vi "Auto_Change _Enum - muti-subvi.vi"() -> ()   [LabVIEW 2015]
uses:
  Enum_Edit Action.ctl
panel:
  in  "製作Form":bool
  in  "初始化歸零?":bool
  out "buttonCluster":T1
  in  "Name_data":string
  in  "Type_Buttom":enum16{"Cluster", "Control"}(ring)=enum."Control"
  in  "Type_Enum":T2(ring)=enum."Constant"
  in  "Value":string[][](array[string])
  in  "Name":string[](array[string])
  in  "檔案格式":enum16{"CSV", "Control"}(ring)
  in  "製作按鈕":bool
  out "Enum":T3
  in  "ReadFromData":bool
  in  "WriteToData":bool
  out "error out":errorcluster
  in  "初始化":bool
  in  "Data":string
  in  "結束":bool
  in  "製作Enum":bool
  in  "儲存CSV":bool
  in  "讀取CSV":bool
  in  "讀取CTL":bool
  in  "error In":errorcluster
  in  "Path":path
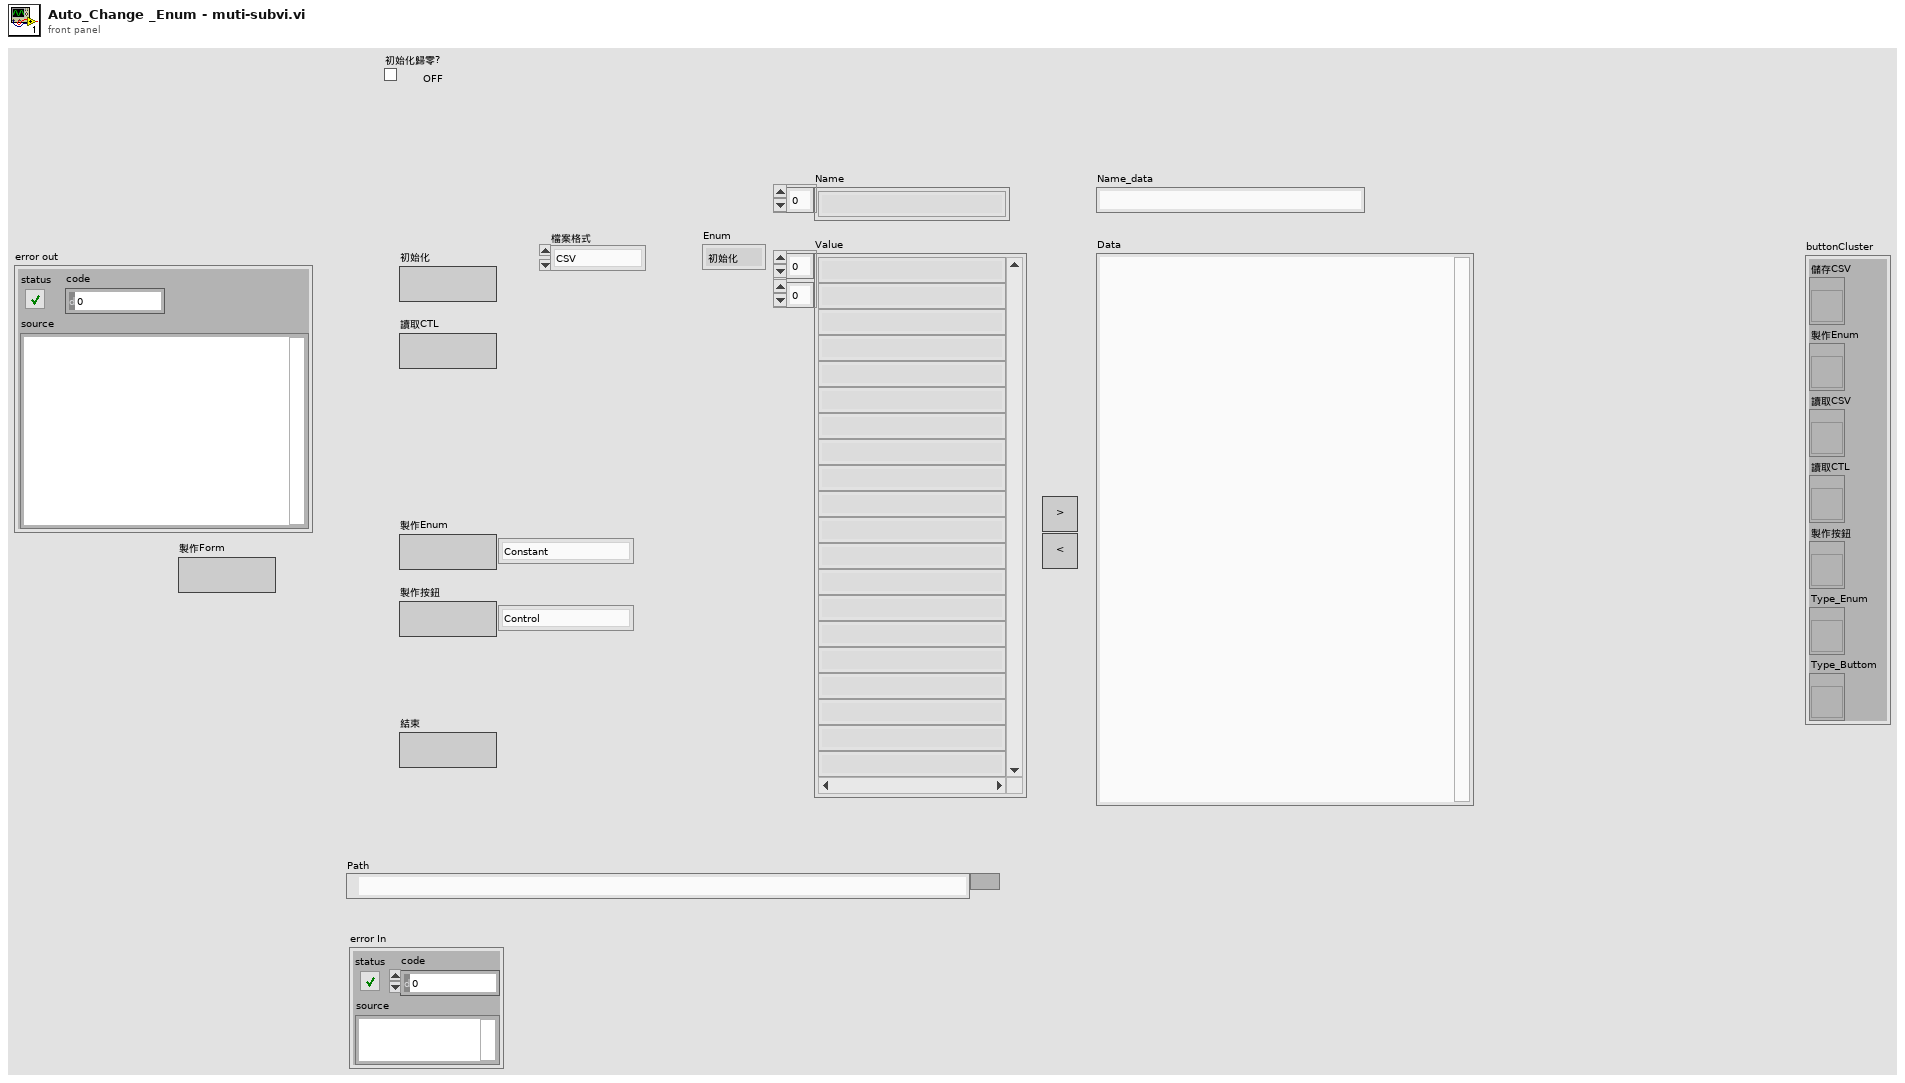
[diagram p1: front panel]
types:
  T1 = cluster{"儲存CSV":refnum<vi>, "製作Enum":refnum<vi>, "讀取CSV":refnum<vi>, "讀取CTL":refnum<vi>, "製作按鈕":refnum<vi>, "Type_Enum":refnum<vi>, "Type_Buttom":refnum<vi>}
  T2 = enum16{"Control", "Constant", "Constant(QMH)", "ClustConstant(QMH)"}
  T3 = typedef "Enum_Edit Action.ctl" = enum16{"初始化", "讀取(CSV)", "讀取(CTL)", "儲存CTL", "儲存CSV", "製作Form", "更新資料", "讀出data區", "寫入data區", "製作按鈕", "閒置", "結束"}
  T4 = cluster{"Alignment":enum32{"Left", "Right", "Hybrid", "Center", "Gravity"}, "Rules":enum32{"Strict", "Allow Wires Under Labels", "Allow Wires Under Lead Nodes", "Allow Wires Under Wide Blocks"}, "Max Heuristic Iterations":u32, "Max Simplex Iterations":u32, "Block Padding":cluster{"Horizontal":i32, "Vertical":i32}, "Wire Padding":cluster{"Horizontal":i32, "Vertical":i32}, "Auto-Tune by Topology":bool, "Fine-Tune Y Positions":bool, "Align All Controls on Left":bool, "Align All Indicators on Right":bool, "Use Array Dimension Heuristics":bool}
  T5 = enum16{"open", "replace", "create", "open or create", "replace or create", "replace or create with confirmation"}
  T6 = enum16{"讀取CTL", "讀取CSV", "儲存CSV", "製作Enum", "製作Form", "結束", "初始化", "Path", "WriteToData", "ReadFromData", "製作按鈕", "檔案格式"}
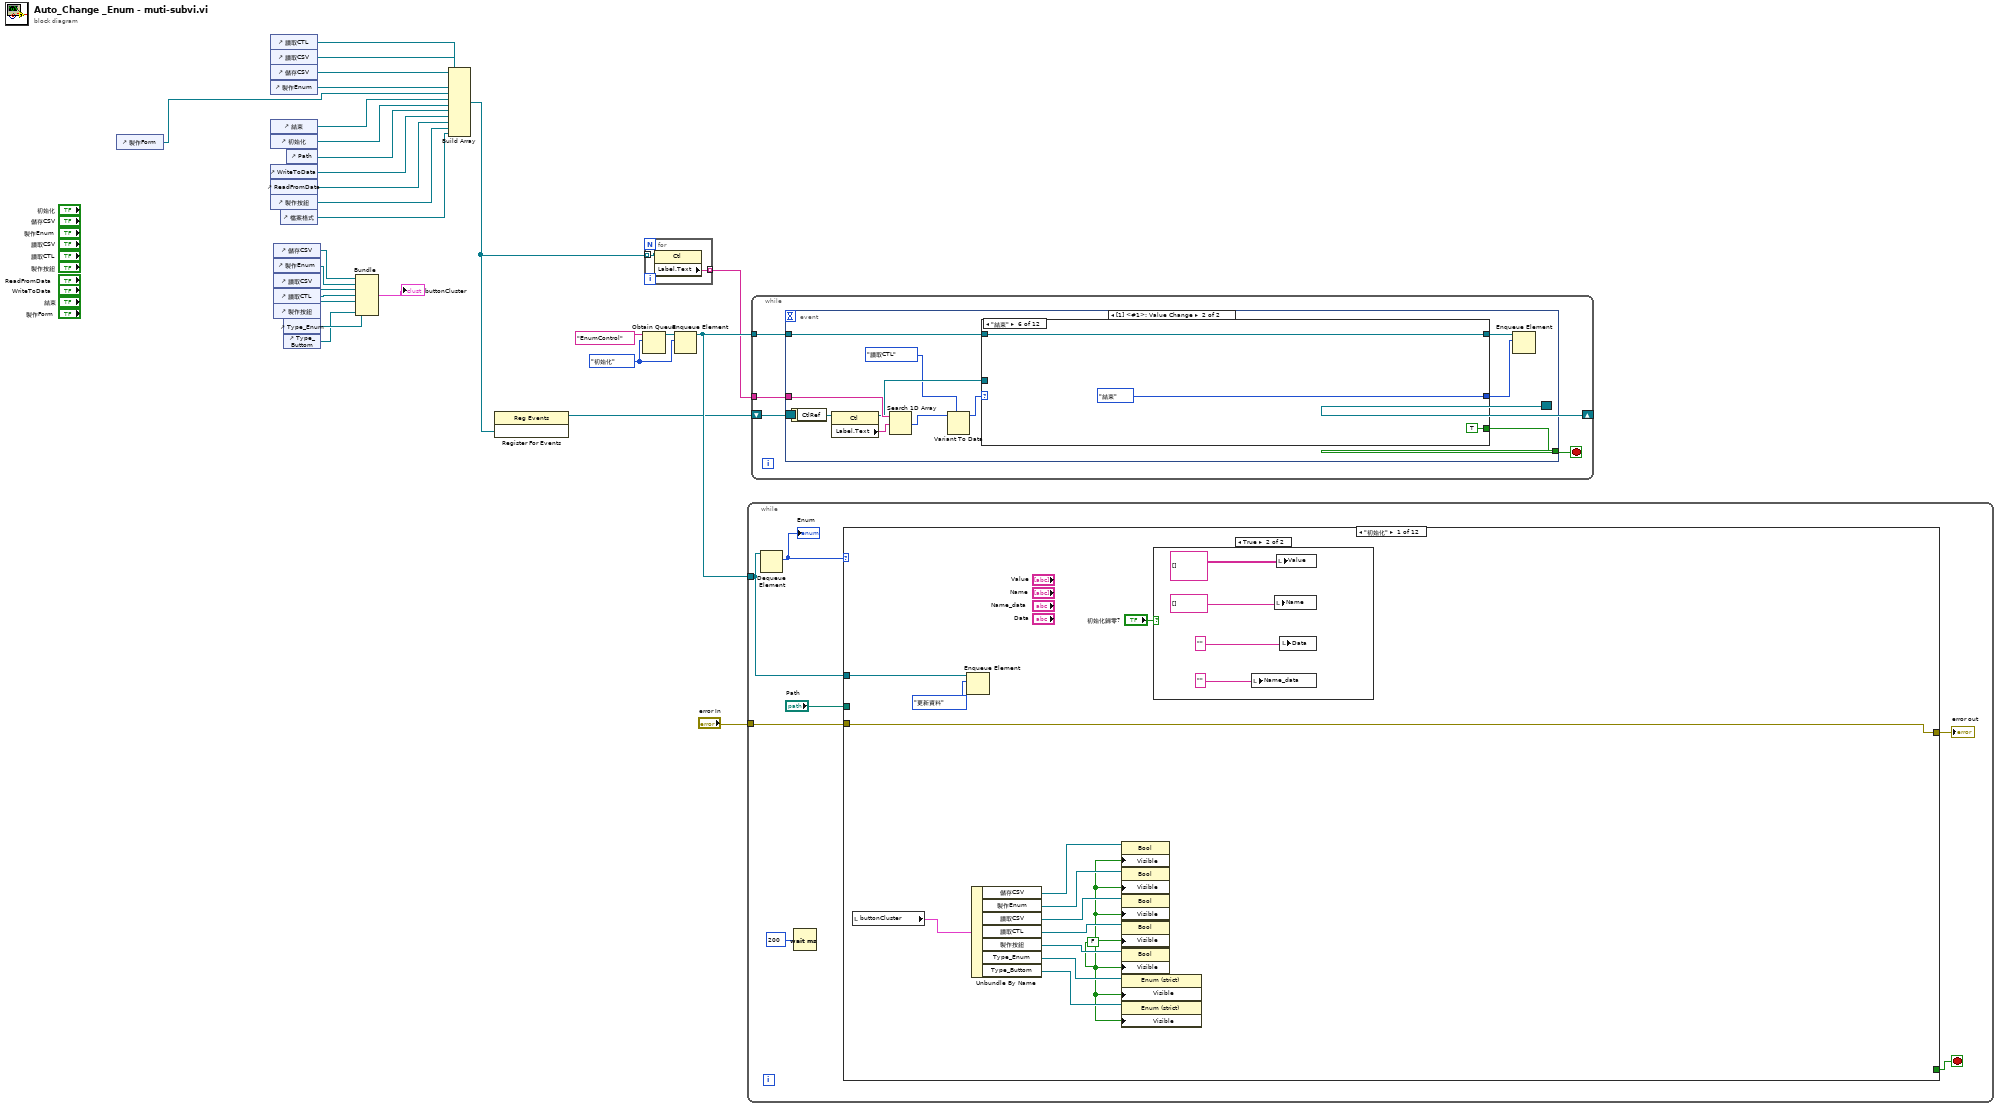
[diagram p0: block diagram]
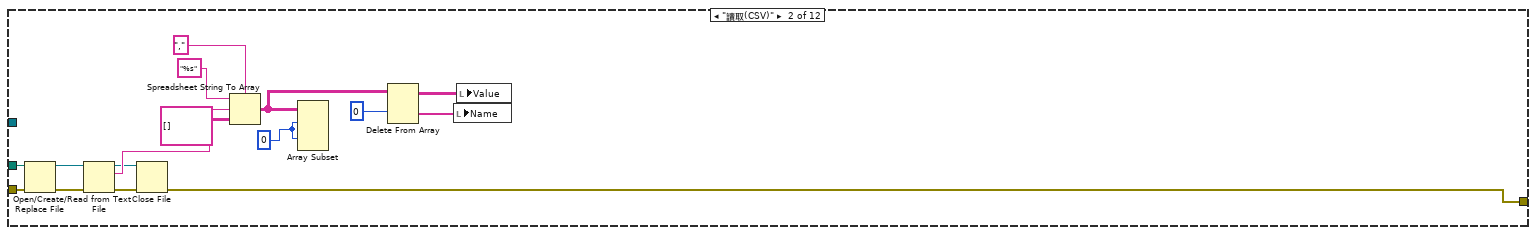
[diagram p3: hidden frame]
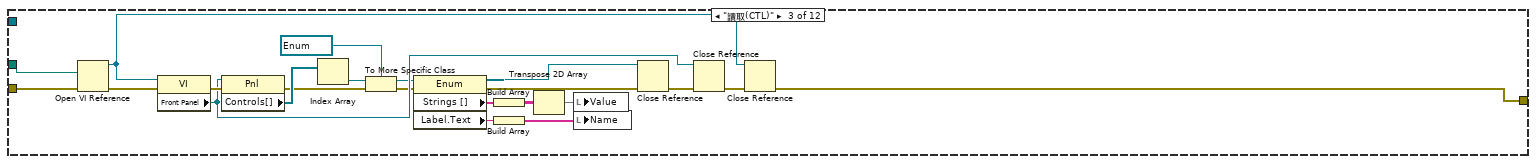
[diagram p4: hidden frame]
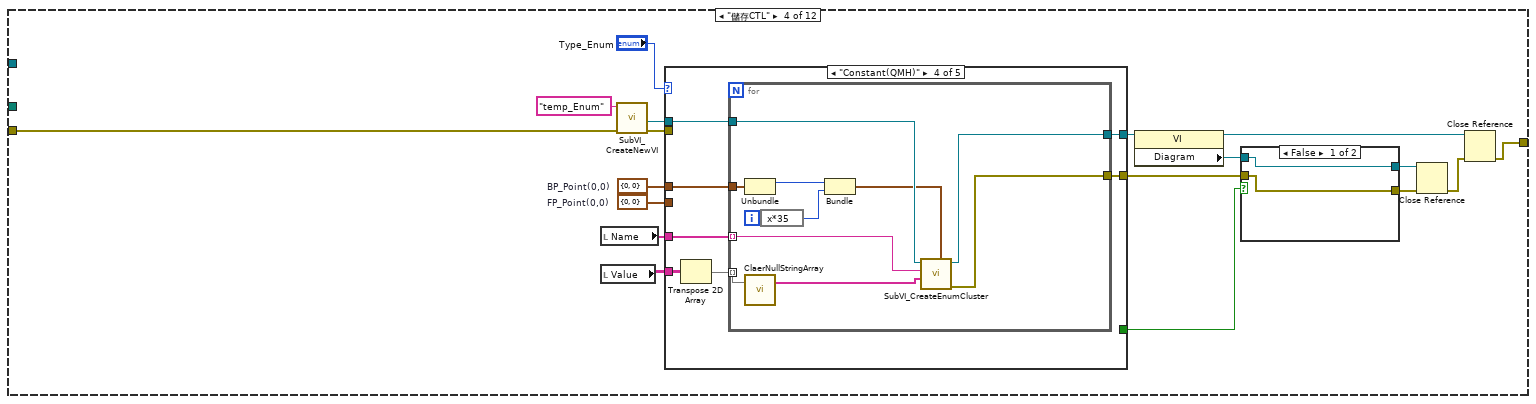
[diagram p5: hidden frame]
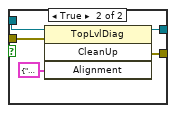
[diagram p6: hidden frame]
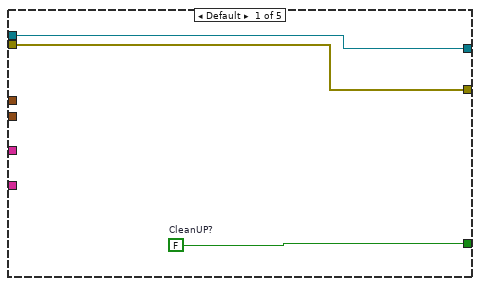
[diagram p7: hidden frame]
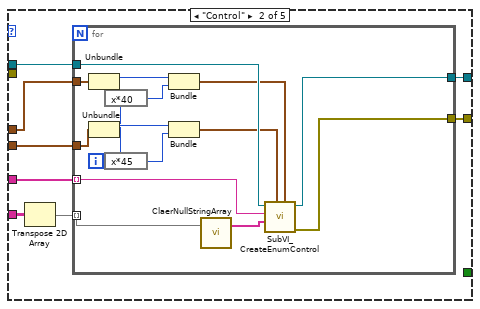
[diagram p8: hidden frame]
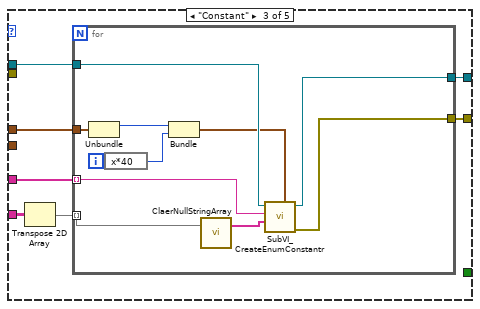
[diagram p9: hidden frame]
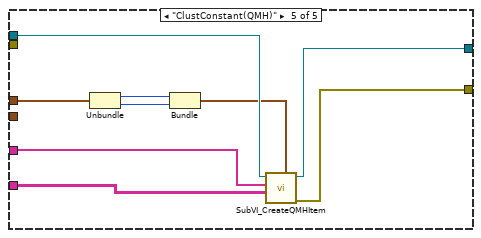
[diagram p10: hidden frame]
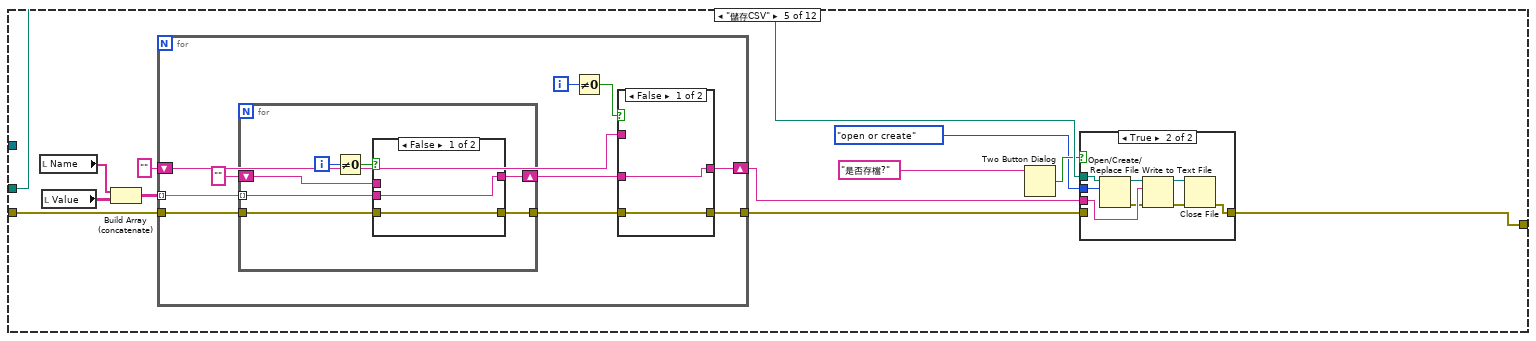
[diagram p11: hidden frame]
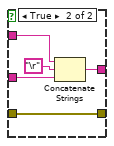
[diagram p13: hidden frame]
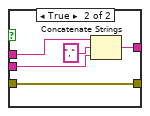
[diagram p14: hidden frame]
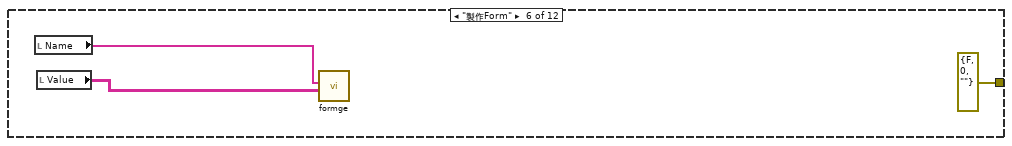
[diagram p15: hidden frame]
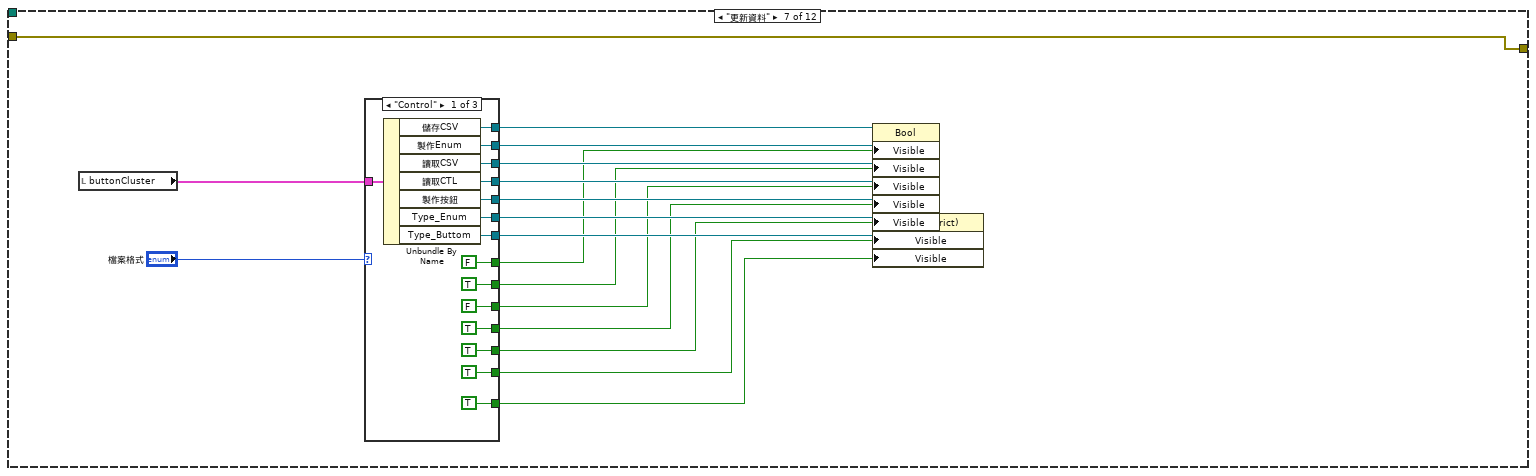
[diagram p16: hidden frame]
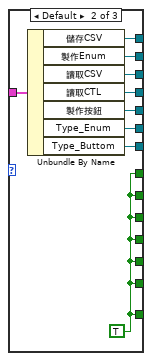
[diagram p17: hidden frame]
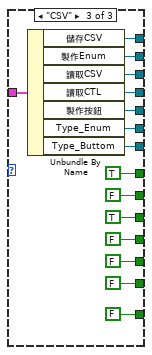
[diagram p18: hidden frame]
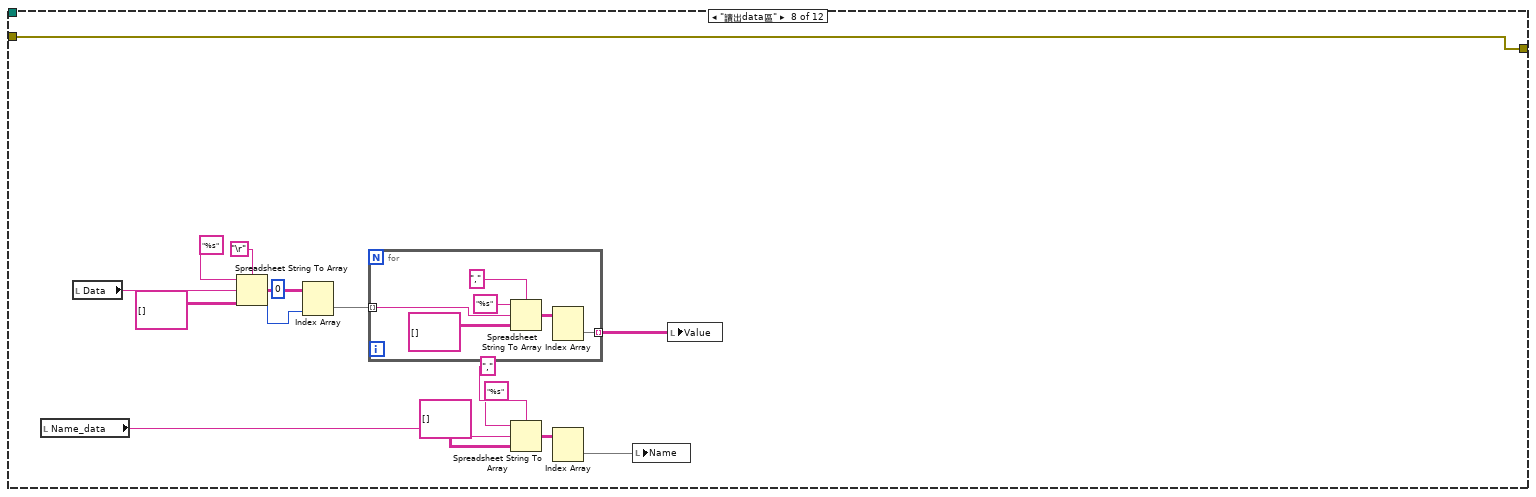
[diagram p19: hidden frame]
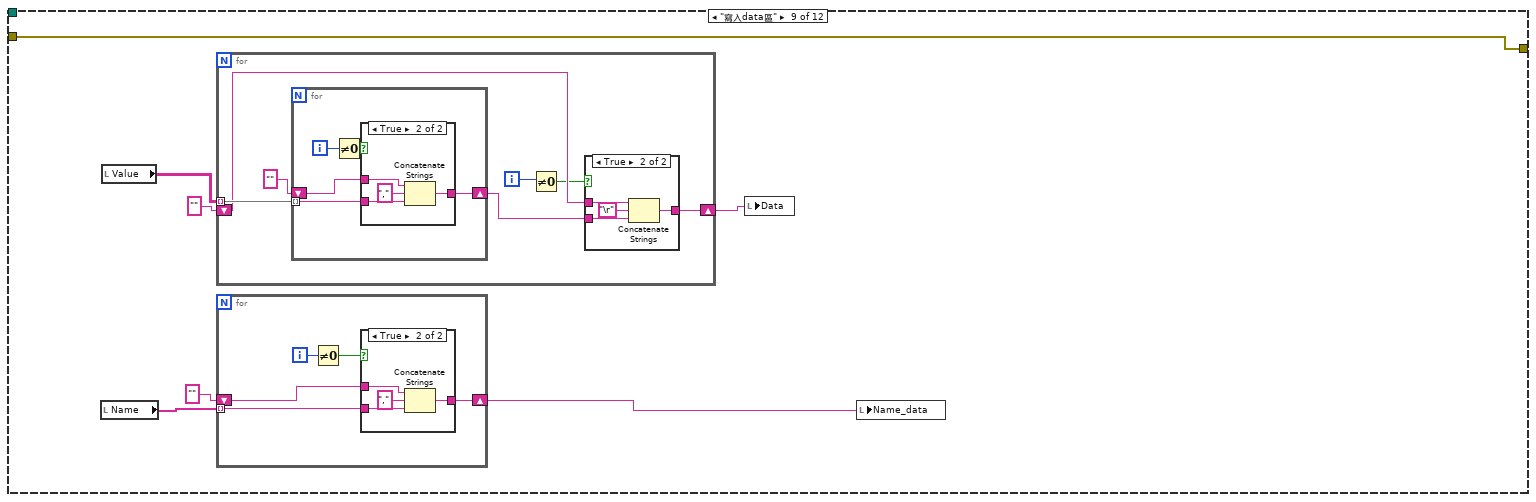
[diagram p20: hidden frame]
diagram:
  w24 = Enum_Edit_Action."初始化" ("Enum")
  n1 = control-ref of="製作Form"() -> (w2:refnum<vi>)
  n2 = control-ref of="讀取CTL"() -> (w15:refnum<vi>)
  n3 = control-ref of="讀取CSV"() -> (w14:refnum<vi>)
  n4 = control-ref of="儲存CSV"() -> (w13:refnum<vi>)
  n5 = control-ref of="製作Enum"() -> (w12:refnum<vi>)
  n6 = control-ref of="結束"() -> (w11:refnum<vi>)
  n7 = control-ref of="初始化"() -> (w10:refnum<vi>)
  n8 = control-ref of="WriteToData"() -> (w8:refnum<vi>)
  n9 = control-ref of="ReadFromData"() -> (w7:refnum<vi>)
  n10 = control-ref of="製作按鈕"() -> (w6:refnum<vi>)
  n11 = control-ref of="儲存CSV"() -> (w21:refnum<vi>)
  n12 = control-ref of="製作Enum"() -> (w16:refnum<vi>)
  n13 = control-ref of="讀取CSV"() -> (w18:refnum<vi>)
  n14 = control-ref of="讀取CTL"() -> (w20:refnum<vi>)
  n15 = control-ref of="製作按鈕"() -> (w19:refnum<vi>)
  n16 = control-ref of="檔案格式"() -> (w5:refnum<vi>)
  n17 = control-ref of="Type_Enum"() -> (w23:refnum<vi>)
  n18 = control-ref of="Type_Buttom"() -> (w17:refnum<vi>)
  n19 = control-ref of="Path"() -> (w9:refnum<vi>)
  n20 = Bundle("儲存CSV"=w21, "製作Enum"=w16, "讀取CSV"=w18, "讀取CTL"=w20, "製作按鈕"=w19, "Type_Enum"=w23, "Type_Buttom"=w17) -> (→"buttonCluster":T1)  [unwired: 1 in]
  n21 = Build Array(w15, w14, w13, w12, w2, w11, w10, w9, w8, w7, w6, w5) -> (w3:refnum<vi>[])
  n22 = register-events(w3) -> (reference out=w22:refnum<event-registration>)  [unwired: 2 in, 1 out]
  n23 = Obtain Queue(name (unnamed)="EnumControl", element data type=w24) -> (queue out=w27:refnum<queue>)  [unwired: 3 in, 2 out]
  n24 = for {
    tunnel: w3 -> [w30] mode=indexing
    tunnel: [w29] -> w1 mode=indexing
    n25 = property class="Ctl"(reference=w30) -> ("Label.Text"=w29:string)  [unwired: 1 in, 2 out]
  }
  n26 = Enqueue Element(queue=w27, element=w24) -> (queue out=w26:refnum<queue>)  [unwired: 2 in, 2 out]
  n27 = while {
    tunnel: w26 -> [w32]
    tunnel: "error In" -> [w35]
    stop <- w36 stop-if-true
    n28 = Dequeue Element(queue=w32) -> (element=w34:T3)  [unwired: 2 in, 3 out]
    "Enum" <- w34
    n29 = Wait (ms)(milliseconds to wait=u32 200) -> ()  [unwired: 1 out]
    n30 = case shown="\"初始化\"" w34 {
      tunnel: [_ _ _ _ _ _ _ _ _ _ _ TRUE] -> w36
      tunnel: w35 -> [w46 w60 w88 w94 w195 _ w260 w314 w327 w372 w440 w441]
      tunnel: [w46 w57 w79 w100 w194 errorcluster {"status"=FALSE, "code"=0, "source"=""} ("error In") w260 w314 w327 w363 w440 w441] -> w33
      tunnel: w32 -> [w43 _ _ _ _ _ _ _ _ _ _ _]
      tunnel: "Path" -> [_ w59 w72 _ w193 _ _ _ _ _ _ _]
      frame "初始化" {
        w39 = FALSE ("Visible")
        n31 = local read "buttonCluster"() -> (w45:T1)
        n32 = Enqueue Element(queue=w43, element=Enum_Edit_Action."更新資料" ("Enum")) -> ()  [unwired: 2 in, 3 out]
        n33 = Unbundle By Name(w45) -> ("儲存CSV"=w50:refnum<vi>, "製作Enum"=w49:refnum<vi>, "讀取CSV"=w48:refnum<vi>, "讀取CTL"=w47:refnum<vi>, "製作按鈕"=w44:refnum<vi>, "Type_Enum"=w41:refnum<vi>, "Type_Buttom"=w40:refnum<vi>)
        n34 = property class="Bool"(reference=w50, "Visible"=w39) -> ()  [unwired: 1 in, 2 out]
        n35 = property class="Bool"(reference=w49, "Visible"=w39) -> ()  [unwired: 1 in, 2 out]
        n36 = property class="Bool"(reference=w48, "Visible"=w39) -> ()  [unwired: 1 in, 2 out]
        n37 = property class="Bool"(reference=w47, "Visible"=w39) -> ()  [unwired: 1 in, 2 out]
        n38 = property class="Bool"(reference=w44, "Visible"=w39) -> ()  [unwired: 1 in, 2 out]
        n39 = property class="Enum (strict)"(reference=w41, "Visible"=w39) -> ()  [unwired: 1 in, 2 out]
        n40 = property class="Enum (strict)"(reference=w40, "Visible"=w39) -> ()  [unwired: 1 in, 2 out]
        n41 = case shown="True" "初始化歸零?" {
          frame False {
          }
          frame True {
            n42 = local write "Name_data"("" ("Data")) -> ()
            n43 = local write "Name"(string[] []) -> ()
            n44 = local write "Value"(string[][] []) -> ()
            n45 = local write "Data"("" ("Data")) -> ()
          }
        }
      }
      frame "讀取(CSV)" {
        w58 = 0 ("index")
        n46 = Open/Create/Replace File(file path (use dialog)=w59, error in=w60) -> (refnum out=w70:refnum<file>, error out=w63:errorcluster)  [unwired: 4 in, 1 out]
        n47 = Read from Text File(file (use dialog)=w70, error in=w63) -> (refnum out=w65:refnum<file>, text=w68:string, error out=w64:errorcluster)  [unwired: 2 in, 1 out]
        n48 = Close File(refnum=w65, error in=w64) -> (error out=w57:errorcluster)  [unwired: 1 out]
        n49 = Spreadsheet String To Array(delimiter (Tab)=",", format string="%s" ("delimiter (\\t)"), spreadsheet string=w68, array type (2D Dbl)=string[][] [] ("Array")) -> (array=w62:string[][])
        n50 = Array Subset(array=w62, index (row)=w58, index (col)=w58) -> ()  [unwired: 2 in, 1 out]
        n51 = Delete From Array(array=w62, index (row)=0) -> (deleted portion=w56:string[], array with subset deleted=w55:string[][])  [unwired: 2 in]
        n52 = local write "Name"(w56) -> ()
        n53 = local write "Value"(w55) -> ()
      }
      frame "讀取(CTL)" {
        n54 = Open VI Reference(vi path=w72, error in (no error)=w88) -> (vi reference=w71:refnum<vi>, error out=w87:errorcluster)  [unwired: 4 in]
        n55 = property class="VI"(reference=w71, error in=w87) -> (error out=w90:errorcluster, "Front Panel"=w89:refnum<vi>)  [unwired: 1 out]
        n56 = property class="Pnl"(reference=w89, error in=w90) -> (error out=w80:errorcluster, "Controls[]"=w86:refnum<vi>[])  [unwired: 1 out]
        n57 = Index Array(array=w86) -> (element=w78:refnum<vi>)  [unwired: 1 in]
        n58 = To More Specific Class(target class=refnum<vi> refnum, reference=w78, error in=w80) -> (specific class reference=w84:refnum<vi>, error out=w82:errorcluster)
        n59 = property class="Enum"(reference=w84, error in=w82) -> (reference out=w83:refnum<vi>, error out=w81:errorcluster, "Strings []"=w77:string[], "Label.Text"=w76:string)
        n60 = Build Array(w77) -> (w74:string[][])
        n61 = Build Array(w76) -> (w75:string[])
        n62 = Transpose 2D Array(2D array=w74) -> (transposed array=w73:string[][])
        n63 = local write "Value"(w73) -> ()
        n64 = local write "Name"(w75) -> ()
        n65 = Close Reference(reference=w83, error in (no error)=w81) -> (error out=w92:errorcluster)
        n66 = Close Reference(reference=w89, error in (no error)=w92) -> (error out=w91:errorcluster)
        n67 = Close Reference(reference=w71, error in (no error)=w91) -> (error out=w79:errorcluster)
      }
      frame "儲存CTL" {
        w97 = cluster{"Width":i32, "Height":i32} {"Width"=0, "Height"=0}  # FP_Point(0,0)
        w98 = cluster{"Width":i32, "Height":i32} {"Width"=0, "Height"=0}  # BP_Point(0,0)
        n68 = local read "Name"() -> (w105:string[])
        n69 = local read "Value"() -> (w110:string[][])
        n70 = call "SubVI_CreateNewVI.vi"("error in (no error)"=w94, "vi path"="temp_Enum") -> ("error out"=w95:errorcluster, "VI out"=w96:refnum<vi>)  [unwired: 8 in]
        n71 = case shown="\"Constant(QMH)\"" "Type_Enum" {
          tunnel: w110 -> [_ w125 w150 w165 w187]
          tunnel: w96 -> [w119 w126 w148 w167 w186]
          tunnel: w105 -> [_ w127 w147 w166 w188]
          tunnel: [w119 w124 w146 w164 w185] -> w104
          tunnel: [w118 w123 w145 w163 w184] -> w101
          tunnel: [w120 _ _ _ _] -> w99
          tunnel: w95 -> [w118 _ _ _ _]
          tunnel: w98 -> [_ w121 w144 w162 w182]
          tunnel: w97 -> [_ w122 _ _ _]
          frame Default {
            w120 = FALSE  # CleanUP?
          }
          frame "Control" {
            n72 = Transpose 2D Array(2D array=w125) -> (transposed array=w128:string[][])
            n73 = for {
              tunnel: w128 -> [w143] mode=indexing
              tunnel: w126 -> [w142]
              tunnel: w127 -> [w139] mode=indexing
              tunnel: [w140] -> w124
              tunnel: [w138] -> w123
              tunnel: w122 -> [w135]
              tunnel: w121 -> [w132]
              i -> [w131]
              n74 = Unbundle(w132) -> ("Width"=w134:i32)  [unwired: 1 out]
              n75 = Unbundle(w135) -> ("Width"=w136:i32)  [unwired: 1 out]
              n76 = expression code="x*40"(w131) -> (w133:i32)
              n77 = expression code="x*45"(w131) -> (w137:i32)
              n78 = Bundle("Width"=w134, w133) -> (w130:cluster{"Width":i32, i32})  [unwired: 1 in]
              n79 = Bundle("Width"=w136, w137) -> (w129:cluster{"Width":i32, i32})  [unwired: 1 in]
              n80 = call <userlib>:"ClaerNullStringArray.vi"("Array in"=w143) -> ("Array out"=w141:string[])  [unwired: 18 in]
              n81 = call "SubVI_CreateEnumControl.vi"("BP_Point(0,0)"=w130, "FP_Point(0,0)"=w129, "Value"=w141, "Name"=w139, "VI in"=w142) -> ("error out"=w138:errorcluster, "VI out"=w140:refnum<vi>)  [unwired: 5 in]
            }
          }
          frame "Constant" {
            n82 = Transpose 2D Array(2D array=w150) -> (transposed array=w149:string[][])
            n83 = for {
              tunnel: w149 -> [w161] mode=indexing
              tunnel: w148 -> [w160]
              tunnel: w147 -> [w157] mode=indexing
              tunnel: [w159] -> w146
              tunnel: [w156] -> w145
              tunnel: w144 -> [w155]
              i -> [w154]
              n84 = Unbundle(w155) -> ("Width"=w151:i32)  [unwired: 1 out]
              n85 = expression code="x*40"(w154) -> (w152:i32)
              n86 = Bundle("Width"=w151, w152) -> (w153:cluster{"Width":i32, i32})  [unwired: 1 in]
              n87 = call <userlib>:"ClaerNullStringArray.vi"("Array in"=w161) -> ("Array out"=w158:string[])  [unwired: 18 in]
              n88 = call "SubVI_CreateEnumConstantr.vi"("BP_Point(0,0)"=w153, "Value"=w158, "Name"=w157, "VI in"=w160) -> ("error out"=w156:errorcluster, "VI out"=w159:refnum<vi>)  [unwired: 6 in]
            }
          }
          frame "Constant(QMH)" {
            n89 = Transpose 2D Array(2D array=w165) -> (transposed array=w168:string[][])
            n90 = for {
              tunnel: w168 -> [w179] mode=indexing
              tunnel: w167 -> [w178]
              tunnel: w166 -> [w177] mode=indexing
              tunnel: [w175] -> w164
              tunnel: [w174] -> w163
              tunnel: w162 -> [w173]
              i -> [w172]
              n91 = Unbundle(w173) -> ("Width"=w169:i32)  [unwired: 1 out]
              n92 = call <userlib>:"ClaerNullStringArray.vi"("Array in"=w179) -> ("Array out"=w176:string[])  [unwired: 18 in]
              n93 = expression code="x*35"(w172) -> (w170:i32)
              n94 = Bundle("Width"=w169, w170) -> (w171:cluster{"Width":i32, i32})  [unwired: 1 in]
              n95 = call "SubVI_CreateEnumCluster.vi"("BP_Point(0,0)"=w171, "Data"=w176, "Name"=w177, "VI in"=w178) -> ("error out"=w174:errorcluster, "VI out"=w175:refnum<vi>)  [unwired: 5 in, 1 out]
            }
          }
          frame "ClustConstant(QMH)" {
            n96 = Unbundle(w182) -> ("Width"=w181:i32, "Height"=w183:i32)
            n97 = Bundle("Width"=w181, "Height"=w183) -> (w180:cluster{"Width":i32, "Height":i32})  [unwired: 1 in]
            n98 = call "SubVI_CreateQMHItem.vi"("BP_Point(0,0)"=w180, "Value"=w187, "Name"=w188, "VI in"=w186) -> ("error out"=w184:errorcluster, "VI out"=w185:refnum<vi>)  [unwired: 6 in]
          }
        }
        n99 = property on="Property Node" class="VI"(reference=w104) -> (reference out=w102:refnum<vi>, "Diagram"=w103:refnum<vi>)  [unwired: 1 in, 1 out]
        n100 = case shown="False" w99 {
          tunnel: [w112 w117] -> w109
          tunnel: [w111 w116] -> w108
          tunnel: w103 -> [w112 w114]
          tunnel: w101 -> [w111 w113]
          frame False {
          }
          frame True {
            n101 = invoke class="TopLvlDiag" method="CleanUp"(reference=w114, error in=w113, "Alignment"=T4 {"Alignment"=enum."Left", "Rules"=enum."Strict", "Max Heuristic Iterations"=0, "Max Simplex Iterations"=0, "Block Padding"={"Horizontal"=0, "Vertical"=0}, "Wire Padding"={"Horizontal"=0, "Vertical"=0}, "Auto-Tune by Topology"=FALSE, "Fine-Tune Y Positions"=FALSE, "Align All Controls on Left"=FALSE, "Align All Indicators on Right"=FALSE, "Use Array Dimension Heuristics"=FALSE} ("Clean Up Options")) -> (reference out=w117:refnum<vi>, error out=w116:errorcluster)  [unwired: 1 in, 2 out]
          }
        }
        n102 = Close Reference(reference=w109, error in (no error)=w108) -> (error out=w107:errorcluster)
        n103 = Close Reference(reference=w102, error in (no error)=w107) -> (error out=w100:errorcluster)
      }
      frame "儲存CSV" {
        n104 = local read "Name"() -> (w197:string[])
        n105 = local read "Value"() -> (w198:string[][])
        n106 = Build Array (concatenate)(w197, w198) -> (w196:string[][])
        n107 = for {
          tunnel: w196 -> [w219] mode=indexing
          shift-right: [w215] -> w200
          shift-left: "" -> [w216]
          tunnel: [w212] -> w199
          tunnel: w195 -> [w210]
          i -> [w214]
          n108 = for {
            tunnel: w219 -> [w233] mode=indexing
            shift-right: [w231] -> w217
            shift-left: "" -> [w232]
            tunnel: [w228] -> w211
            tunnel: w210 -> [w227]
            i -> [w230]
            n109 = Not Equal To 0?(x=w230) -> (x != 0?=w229:bool)
            n110 = case shown="False" w229 {
              tunnel: w233 -> [w235 w239]
              tunnel: w232 -> [_ w238]
              tunnel: [w235 w237] -> w231
              tunnel: [w234 w236] -> w228
              tunnel: w227 -> [w234 w236]
              frame False {
              }
              frame True {
                n111 = Concatenate Strings(w238, ",", w239) -> (w237:string)
              }
            }
          }
          n112 = Not Equal To 0?(x=w214) -> (x != 0?=w213:bool)
          n113 = case shown="False" w213 {
            tunnel: w217 -> [w221 w226]
            tunnel: w216 -> [_ w224]
            tunnel: [w221 w223] -> w215
            tunnel: [w220 w222] -> w212
            tunnel: w211 -> [w220 w222]
            frame False {
            }
            frame True {
              n114 = Concatenate Strings(w224, "\r", w226) -> (w223:string)
            }
          }
        }
        n115 = Two Button Dialog(message="是否存檔?") -> (T button?=w191:bool)  [unwired: 2 in]
        n116 = case shown="True" w191 {
          tunnel: T5."open or create" ("operation (0:open)") -> [_ w208]
          tunnel: w200 -> [_ w207]
          tunnel: [w201 w204] -> w194
          tunnel: w193 -> [_ w202]
          tunnel: w199 -> [w201 _]
          frame False {
          }
          frame True {
            n117 = Open/Create/Replace File(file path (use dialog)=w202, operation (0:open)=w208) -> (refnum out=w209:refnum<file>, error out=w203:errorcluster)  [unwired: 4 in, 1 out]
            n118 = Write to Text File(file (use dialog)=w209, text=w207, error in=w203) -> (refnum out=w205:refnum<file>, error out=w206:errorcluster)  [unwired: 1 in, 1 out]
            n119 = Close File(refnum=w205, error in=w206) -> (error out=w204:errorcluster)  [unwired: 1 out]
          }
        }
      }
      frame "製作Form" {
        n120 = local read "Name"() -> (w242:string[])
        n121 = local read "Value"() -> (w241:string[][])
        n122 = call "formge.vi"("Data"=w241, "DataName"=w242) -> ()  [unwired: 10 in]
      }
      frame "更新資料" {
        n123 = local read "buttonCluster"() -> (w247:T1)
        n124 = case shown="\"Control\"" "檔案格式" {
          tunnel: w247 -> [w268 w276 w299]
          tunnel: [w275 w284 w298] -> w259
          tunnel: [w274 w283 w297] -> w258
          tunnel: [w273 w282 w296] -> w257
          tunnel: [w272 w281 w295] -> w256
          tunnel: [w271 w280 w294] -> w255
          tunnel: [w270 w279 w293] -> w254
          tunnel: [w269 w278 w292] -> w253
          tunnel: [TRUE ("Visible") w277 FALSE ("Visible")] -> w252
          tunnel: [TRUE ("Visible") w277 FALSE ("Visible")] -> w244
          tunnel: [TRUE ("Visible") w277 FALSE ("Visible")] -> w251
          tunnel: [FALSE ("Visible") w277 TRUE ("Visible")] -> w250
          tunnel: [TRUE ("Visible") w277 FALSE ("Visible")] -> w249
          tunnel: [FALSE ("Visible") w277 TRUE ("Visible")] -> w248
          tunnel: [TRUE ("Visible") w277 FALSE ("Visible")] -> w245
          frame "Control" {
            n125 = Unbundle By Name(w268) -> ("儲存CSV"=w275:refnum<vi>, "製作Enum"=w274:refnum<vi>, "讀取CSV"=w273:refnum<vi>, "讀取CTL"=w272:refnum<vi>, "製作按鈕"=w271:refnum<vi>, "Type_Enum"=w270:refnum<vi>, "Type_Buttom"=w269:refnum<vi>)
          }
          frame Default {
            w277 = TRUE ("Visible")
            n126 = Unbundle By Name(w276) -> ("儲存CSV"=w284:refnum<vi>, "製作Enum"=w283:refnum<vi>, "讀取CSV"=w282:refnum<vi>, "讀取CTL"=w281:refnum<vi>, "製作按鈕"=w280:refnum<vi>, "Type_Enum"=w279:refnum<vi>, "Type_Buttom"=w278:refnum<vi>)
          }
          frame "CSV" {
            n127 = Unbundle By Name(w299) -> ("儲存CSV"=w298:refnum<vi>, "製作Enum"=w297:refnum<vi>, "讀取CSV"=w296:refnum<vi>, "讀取CTL"=w295:refnum<vi>, "製作按鈕"=w294:refnum<vi>, "Type_Enum"=w293:refnum<vi>, "Type_Buttom"=w292:refnum<vi>)
          }
        }
        n128 = property class="Bool"(reference=w259, "Visible"=w248) -> ()  [unwired: 1 in, 2 out]
        n129 = property class="Bool"(reference=w258, "Visible"=w249) -> ()  [unwired: 1 in, 2 out]
        n130 = property class="Bool"(reference=w257, "Visible"=w250) -> ()  [unwired: 1 in, 2 out]
        n131 = property class="Bool"(reference=w256, "Visible"=w245) -> ()  [unwired: 1 in, 2 out]
        n132 = property class="Bool"(reference=w255, "Visible"=w251) -> ()  [unwired: 1 in, 2 out]
        n133 = property class="Enum (strict)"(reference=w254, "Visible"=w244) -> ()  [unwired: 1 in, 2 out]
        n134 = property class="Enum (strict)"(reference=w253, "Visible"=w252) -> ()  [unwired: 1 in, 2 out]
      }
      frame "讀出data區" {
        n135 = local read "Name_data"() -> (w302:string)
        n136 = local read "Data"() -> (w307:string)
        n137 = Spreadsheet String To Array(delimiter (Tab)="\r", format string="%s", spreadsheet string=w307, array type (2D Dbl)=string[][] []) -> (array=w312:string[][])
        n138 = Index Array(array=w312, index (col)=0 ("disabled index (col)")) -> (element=w309:string[])  [unwired: 1 in]
        n139 = for {
          tunnel: w309 -> [w318] mode=indexing
          tunnel: [w316] -> w308 mode=indexing
          n140 = Spreadsheet String To Array(delimiter (Tab)="," ("format string"), format string="%s", spreadsheet string=w318, array type (2D Dbl)=string[][] []) -> (array=w315:string[][])
          n141 = Index Array(array=w315) -> (element=w316:string[])  [unwired: 2 in]
        }
        n142 = Spreadsheet String To Array(delimiter (Tab)="," ("format string"), format string="%s", spreadsheet string=w302, array type (2D Dbl)=string[][] []) -> (array=w306:string[][])
        n143 = Index Array(array=w306) -> (element=w301:string[])  [unwired: 2 in]
        n144 = local write "Name"(w301) -> ()
        n145 = local write "Value"(w308) -> ()
      }
      frame "寫入data區" {
        n146 = local read "Name"() -> (w323:string[])
        n147 = local read "Value"() -> (w324:string[][])
        n148 = for {
          tunnel: w324 -> [w344] mode=indexing
          shift-right: [w340] -> w325
          shift-left: "" -> [w341]
          i -> [w339]
          n149 = for {
            tunnel: w344 -> [w354] mode=indexing
            shift-right: [w352] -> w342
            shift-left: "" -> [w353]
            i -> [w350]
            n150 = Not Equal To 0?(x=w350) -> (x != 0?=w351:bool)
            n151 = case shown="True" w351 {
              tunnel: w354 -> [w355 w358]
              tunnel: w353 -> [_ w356]
              tunnel: [w355 w357] -> w352
              frame False {
              }
              frame True {
                n152 = Concatenate Strings(w356, ",", w358) -> (w357:string)
              }
            }
          }
          n153 = Not Equal To 0?(x=w339) -> (x != 0?=w338:bool)
          n154 = case shown="True" w338 {
            tunnel: w342 -> [w345 w349]
            tunnel: w341 -> [_ w347]
            tunnel: [w345 w346] -> w340
            frame False {
            }
            frame True {
              n155 = Concatenate Strings(w347, "\r", w349) -> (w346:string)
            }
          }
        }
        n156 = for {
          tunnel: w323 -> [w332] mode=indexing
          shift-right: [w330] -> w321
          shift-left: "" -> [w331]
          i -> [w328]
          n157 = Not Equal To 0?(x=w328) -> (x != 0?=w329:bool)
          n158 = case shown="True" w329 {
            tunnel: w332 -> [w333 w336]
            tunnel: w331 -> [_ w334]
            tunnel: [w333 w335] -> w330
            frame False {
            }
            frame True {
              n159 = Concatenate Strings(w334, ",", w336) -> (w335:string)
            }
          }
        }
        n160 = local write "Data"(w325) -> ()
        n161 = local write "Name_data"(w321) -> ()
      }
      frame "製作按鈕" {
        w370 = cluster{"Width":i32, "Height":i32} {"Width"=0, "Height"=0}  # BP_Point(0,0)
        w371 = cluster{"Width":i32, "Height":i32} {"Width"=0, "Height"=0}  # FP_Point(0,0)
        n162 = local read "Name"() -> (w375:string[])
        n163 = local read "Value"() -> (w374:string[][])
        n164 = Transpose 2D Array(2D array=w374) -> (transposed array=w373:string[][])
        n165 = call "SubVI_CreateNewVI.vi"("error in (no error)"=w372, "vi path"="temp_Buttom") -> ("error out"=w377:errorcluster, "VI out"=w379:refnum<vi>)  [unwired: 8 in]
        n166 = for {
          tunnel: w379 -> [w395]
          tunnel: w377 -> [w397]
          tunnel: [w396] -> w362
          tunnel: w373 -> [w393] mode=indexing
          tunnel: w375 -> [w394] mode=indexing
          tunnel: "Type_Buttom" -> [w391]
          tunnel: w371 -> [w390]
          tunnel: w370 -> [w389]
          tunnel: [w388] -> w368
          tunnel: [w387] -> w360
          i -> [w392]
          n167 = case shown="\"Cluster\"" w391 {
            tunnel: w397 -> [w408 w418 w439]
            tunnel: [w412 w418 w429] -> w396
            tunnel: w395 -> [w411 w419 w427]
            tunnel: w394 -> [w414 _ _]
            tunnel: w393 -> [w417 _ w438]
            tunnel: w392 -> [w403 _ w437]
            tunnel: w390 -> [w399 _ w421]
            tunnel: w389 -> [w400 _ w423]
            tunnel: [w410 w419 w426] -> w388
            tunnel: [_ w420 _] -> w387
            frame "Cluster" {
              n168 = call <userlib>:"ClaerNullStringArray.vi"("Array in"=w417) -> ("Array out"=w415:string[])  [unwired: 18 in]
              n169 = expression code="x*110"(w403) -> (w405:i32)
              n170 = Bundle(w405, 0) -> (w404:cluster{i32, i32})  [unwired: 1 in]
              n171 = Add(x=w404, y=w400) -> (x+y=w401:cluster{i32, i32})
              n172 = Add(x=w404, y=w399) -> (x+y=w398:cluster{i32, i32})
              n173 = call "SubVI_CreateBottomCluster.vi"("BP_Point(0,0)"=w401, "FP_Point(0,0)"=w398, "error in (no error)"=w408, "Value"=w415, "Name"=w414, "VI in"=w411) -> ("error out"=w409:errorcluster, "Array"=w413:refnum<vi>[], "VI out"=w416:refnum<vi>)  [unwired: 3 in]
              n174 = Add(x=w401, y=cluster{"Width":i32, "Height":i32} {"Width"=1200, "Height"=100}) -> (x+y=w406:cluster{i32, i32})
              n175 = call "SubVI_CreateBuildArray.vi"("BP_Point(0,0)"=w406, "error in (no error)"=w409, "Array"=w413, "VI in"=w416) -> ("error out"=w412:errorcluster, "VI out"=w410:refnum<vi>)  [unwired: 5 in, 1 out]
            }
            frame Default {
              w420 = FALSE  # CleanUP?
            }
            frame "Control" {
              n176 = call <userlib>:"ClaerNullStringArray.vi"("Array in"=w438) -> ("Array out"=w435:string[])  [unwired: 18 in]
              n177 = expression code="x*110"(w437) -> (w436:i32)
              n178 = Bundle(w436, 0) -> (w422:cluster{i32, i32})  [unwired: 1 in]
              n179 = Add(x=w422, y=w423) -> (x+y=w425:cluster{i32, i32})
              n180 = Add(x=w422, y=w421) -> (x+y=w424:cluster{i32, i32})
              n181 = call "SubVI_CreateBottom.vi"("BP_Point(0,0)"=w425, "FP_Point(0,0)"=w424, "error in (no error)"=w439, "Value"=w435, "VI in"=w427) -> ("error out"=w430:errorcluster, "Array"=w433:refnum<vi>[], "VI out"=w434:refnum<vi>)  [unwired: 4 in]
              n182 = Add(x=w425, y=cluster{i32, i32} {1200, 100}) -> (x+y=w431:cluster{i32, i32})
              n183 = call "SubVI_CreateBuildArray.vi"("BP_Point(0,0)"=w431, "error in (no error)"=w430, "Array"=w433, "VI in"=w434) -> ("error out"=w429:errorcluster, "VI out"=w426:refnum<vi>)  [unwired: 5 in, 1 out]
            }
          }
        }
        n184 = property on="Property Node" class="VI"(reference=w368, error in=w362) -> (reference out=w369:refnum<vi>, error out=w366:errorcluster, "Diagram"=w367:refnum<vi>)
        n185 = case shown="True" w360 {
          tunnel: w367 -> [w381 w385]
          tunnel: w366 -> [w380 w384]
          tunnel: [w380 w383] -> w365
          tunnel: [w381 w382] -> w361
          frame False {
          }
          frame True {
            n186 = invoke class="TopLvlDiag" method="CleanUp"(reference=w385, error in=w384, "Alignment"=T4 {"Alignment"=enum."Left", "Rules"=enum."Strict", "Max Heuristic Iterations"=0, "Max Simplex Iterations"=0, "Block Padding"={"Horizontal"=0, "Vertical"=0}, "Wire Padding"={"Horizontal"=0, "Vertical"=0}, "Auto-Tune by Topology"=FALSE, "Fine-Tune Y Positions"=FALSE, "Align All Controls on Left"=TRUE, "Align All Indicators on Right"=TRUE, "Use Array Dimension Heuristics"=FALSE} ("Clean Up Options")) -> (reference out=w382:refnum<vi>, error out=w383:errorcluster)  [unwired: 1 in, 2 out]
          }
        }
        n187 = Close Reference(reference=w361, error in (no error)=w365) -> (error out=w364:errorcluster)
        n188 = Close Reference(reference=w369, error in (no error)=w364) -> (error out=w363:errorcluster)
      }
      frame "閒置", Default {
      }
      frame "結束" {
      }
    }
    "error out" <- w33
  }
  n189 = while {
    tunnel: w26 -> [w447]
    tunnel: w1 -> [w444]
    shift-right: [w443] -> _
    shift-left: w22 -> [w445]
    stop <- w446 stop-if-true
    n190 = event shown="[1] <#1>: Value Change" {
      selector: w445 -> [_ _]
      dyn-events: [_ _] -> w443
      timeout: _ -> [_ _]
      tunnel: w447 -> [_ w454]
      tunnel: [_ w449] -> w446
      tunnel: w444 -> [_ w457]
      event Timeout {
        n191 = event-data() -> ()  [unwired: 1 in, 3 out]
      }
      event Value Change {
        n192 = event-data() -> ("CtlRef"=w458:refnum<vi>)  [unwired: 1 in]
        n193 = property class="Ctl"(reference=w458) -> (reference out=w450:refnum<vi>, "Label.Text"=w456:string)  [unwired: 1 in, 1 out]
        n194 = Search 1D Array(1D array=w457, element=w456) -> (index of element=w455:i32)  [unwired: 1 in]
        n195 = Variant To Data(type=T6."讀取CTL", Variant=w455) -> (data=w453:T6)  [unwired: 1 in, 1 out]
        n196 = case shown="\"結束\"" w453 {
          tunnel: w454 -> [w461 w463 w465 w467 w469 w472 w474 w483 w487 w489 w491 w493]
          tunnel: [w461 w463 w465 w467 w469 w472 w474 w483 w487 w489 w491 w493] -> w452
          tunnel: [Enum_Edit_Action."讀取(CTL)" ("Enum") Enum_Edit_Action."讀取(CSV)" ("Enum") Enum_Edit_Action."儲存CSV" ("Enum") Enum_Edit_Action."儲存CTL" ("Enum") Enum_Edit_Action."製作Form" ("Enum") Enum_Edit_Action."結束" ("Enum") Enum_Edit_Action."初始化" ("Enum") Enum_Edit_Action."更新資料" ("Enum") Enum_Edit_Action."寫入data區" ("Enum") Enum_Edit_Action."讀出data區" ("Enum") Enum_Edit_Action."製作按鈕" ("Enum") Enum_Edit_Action."更新資料" ("Enum")] -> w451
          tunnel: w450 -> [_ _ _ _ _ _ _ w481 _ _ _ _]
          tunnel: [FALSE _ _ _ _ TRUE _ _ _ _ _ _] -> w449
          frame "讀取CTL", Default {
          }
          frame "讀取CSV" {
          }
          frame "儲存CSV" {
          }
          frame "製作Enum" {
          }
          frame "製作Form" {
          }
          frame "結束" {
          }
          frame "初始化" {
          }
          frame "Path" {
            n197 = property class="Ctl"(reference=w481) -> ("Value"=w480:variant)  [unwired: 1 in, 2 out]
            n198 = Variant To Data(type=path "", Variant=w480) -> (data=w476:path)  [unwired: 1 in, 1 out]
            n199 = Strip Path(path=w476) -> (name=w478:string)  [unwired: 1 out]
            n200 = Search/Split String(string=w478, search string/char (-)="." ("regular expression")) -> (match + rest of string=w475:string)  [unwired: 1 in, 2 out]
            n201 = case shown="\".ctl\"" w475 {
              frame ".ctl" {
                n202 = local write "檔案格式"(enum16{"CSV", "Control"}."Control" ("檔案格式")) -> ()
              }
              frame Default {
              }
              frame ".csv" {
                n203 = local write "檔案格式"(enum16{"CSV", "Control"}."CSV" ("檔案格式")) -> ()
              }
            }
          }
          frame "WriteToData" {
          }
          frame "ReadFromData" {
          }
          frame "製作按鈕" {
          }
          frame "檔案格式" {
          }
        }
        n204 = Enqueue Element(queue=w452, element=w451) -> ()  [unwired: 2 in, 3 out]
      }
    }
  }
